vi "Grid_Data.vi"(2 "Transpose":bool, 3 "XY Graph":cluster{dbl[], dbl[]}[](array[cluster]) {"?" format="%.2f"; "?" format="%.2f"}, 4 "Bin Centres":dbl[](array[numeric]) format="%.2f") -> (0 "No of Duplicates":i32, 1 "Grided data":dbl[][](array[numeric]) format="%.2f")   [LabVIEW 2010]
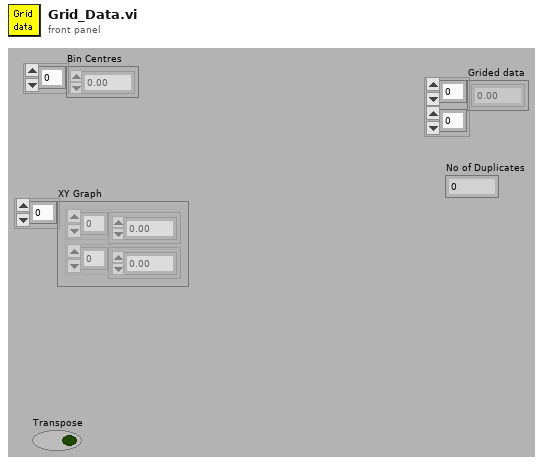
[diagram p1: front panel]
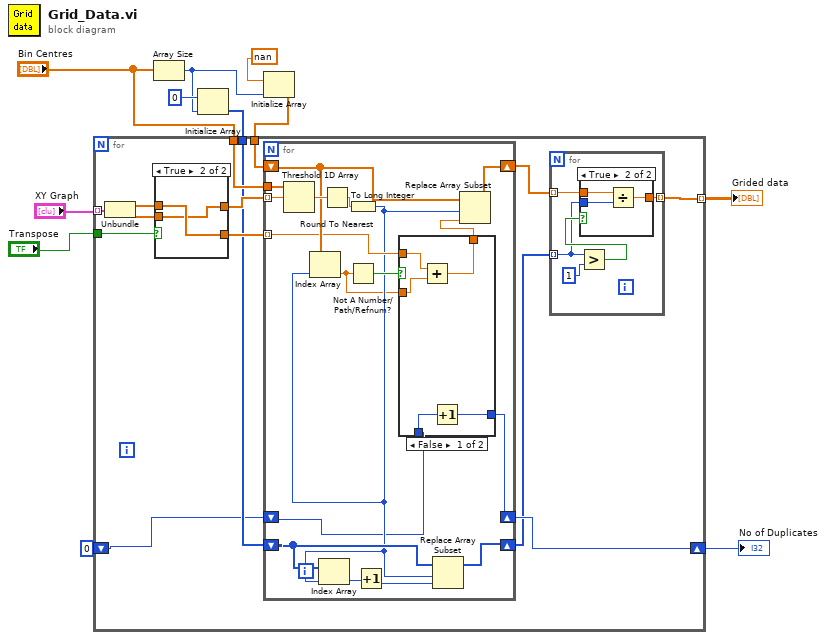
[diagram p0: block diagram]
diagram:
  n1 = Array Size(array="Bin Centres") -> (size(s)=w9:i32)
  n2 = Initialize Array(0 ("element"), w9) -> (w11:i32[])
  n3 = Initialize Array(nan, w9) -> (w4:dbl[])
  n4 = for {
    tunnel: "XY Graph" -> [w25] mode=indexing
    tunnel: "Transpose" -> [w24]
    tunnel: "Bin Centres" -> [w22]
    tunnel: w4 -> [w18]
    shift-right: [w15] -> w8
    shift-left: 0 -> [w16]
    tunnel: w11 -> [w17]
    tunnel: [w12] -> w1 mode=indexing
    n5 = Unbundle(w25) -> (w23:dbl[], w20:dbl[])
    n6 = case shown="True" w24 {
      tunnel: [w60 w61] -> w21
      tunnel: w23 -> [w60 w62]
      tunnel: w20 -> [w59 w61]
      tunnel: [w59 w62] -> w19
      frame False {
      }
      frame True {
      }
    }
    n7 = for {
      tunnel: w22 -> [w51]
      tunnel: w21 -> [w50] mode=indexing
      tunnel: w19 -> [w40] mode=indexing
      shift-right: [w47] -> w13
      shift-left: w18 -> [w42]
      shift-right: [w43] -> w14
      shift-left: w17 -> [w44]
      shift-right: [w35] -> w15
      shift-left: w16 -> [w36]
      n8 = Threshold 1D Array(2:w50, 3:w51) -> (0:w49:dbl)  [unwired: 1 out]
      n9 = Round To Nearest(number=w49) -> (nearest integer value=w48:dbl)
      n10 = To Long Integer(number=w48) -> (32bit integer=w39:i32)
      n11 = Index Array(array=w42, index=w39) -> (element=w37:dbl)
      n12 = Index Array(array=w44, index=w39) -> (element=w46:i32)
      n13 = Not A Number/Path/Refnum?(number/path/refnum=w37) -> (NaN/Path/Refnum?=w41:bool)
      n14 = Increment(x=w46) -> (x+1=w45:i32)
      n15 = case shown="False" w41 {
        tunnel: [w55 w58] -> w38
        tunnel: w40 -> [w52 w58]
        tunnel: w37 -> [w56 _]
        tunnel: w36 -> [w54 w57]
        tunnel: [w53 w57] -> w35
        frame False {
          n16 = Add(x=w52, y=w56) -> (x+y=w55:dbl)
          n17 = Increment(x=w54) -> (x+1=w53:i32)
        }
        frame True {
        }
      }
      n18 = Replace Array Subset(array=w44, new element=w45, index=w39) -> (w43:i32[])
      n19 = Replace Array Subset(array=w42, new element=w38, index=w39) -> (w47:dbl[])
    }
    n20 = for {
      tunnel: w14 -> [w27] mode=indexing
      tunnel: w13 -> [w28] mode=indexing
      tunnel: [w26] -> w12 mode=indexing
      n21 = Greater?(x=w27, y=1) -> (0:w29:bool)
      n22 = case shown="True" w29 {
        tunnel: w28 -> [w31 w34]
        tunnel: w27 -> [_ w33]
        tunnel: [w31 w32] -> w26
        frame False {
        }
        frame True {
          n23 = Divide(x=w34, y=w33) -> (x/y=w32:dbl)
        }
      }
    }
  }
  "No of Duplicates" <- w8
  "Grided data" <- w1
